vi "MOCKBEAR_Resample.vi"(8 "error in (no error)":errorcluster, 10 "FEA_Model in":refnum<class "FEA_Model.lvclass">, 11 "MOCKBEAR in":refnum<class "MOCKBEAR.lvclass">) -> (0 "error out":errorcluster, 3 "MOCKBEAR out":refnum<class "MOCKBEAR.lvclass">)   [LabVIEW 2021, in "MOCKBEAR.lvclass"]
uses:
  MOCKBEAR.lvclass
  FEA_Model/FEA_Model.lvclass
  MOCKBEAR.lvclass/MOCKBEAR.ctl
panel:
  in  "FFT Window":i32
  in  "New sample rate":dbl
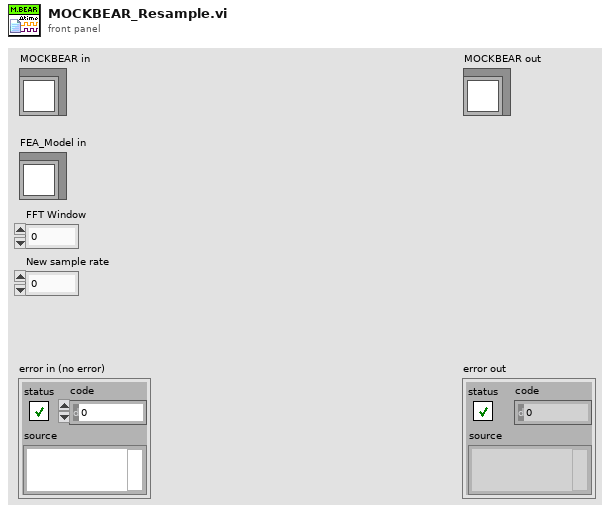
[diagram p1: front panel]
types:
  T1 = enum16{"Recorded", "Auto Resample", "Custom Resample"}
  T2 = cluster{"Modeling Parameters":cluster{"beam_length":dbl, "youngs_modulus":dbl, "torsion_spring":dbl, "beam_height":dbl, "beam_width":dbl, "beam_density":dbl, "number_of_FEA_nodes":i32, "accelerometer_mass":dbl, "M Matrix":dbl[][], "K Matrix":dbl[][], "nodes_of_interest":i32[], "all_nodes":i32[]}, "Simulation Parameters":cluster{"Eigensolver ":enum16{"LabVIEW Cholesky", "LabVIEW General", "LabVIEW Inverse", "LEMP"}, "Pin Estimate":i32, "Frequency Estimate":dbl, "Models Forcasted":i32, "Max frequency":dbl, "Min frequency":dbl, "Frequency delta per node":dbl, "Max frequency delta per second":dbl, "Max Roller Velocity":dbl, "Max Roller Position Percent":dbl, "Min Roller Position Percent":dbl, "Particle Frequencies":dbl[], "Particles":i32[], "Particles Positions":dbl[], "Frequency Target":dbl, "Position estimate":dbl}, "LEMP":cluster{"Eigenvalues":dbl[], "SquareT Eigenvectors":dbl[][], "1/deltaStiff":dbl}}
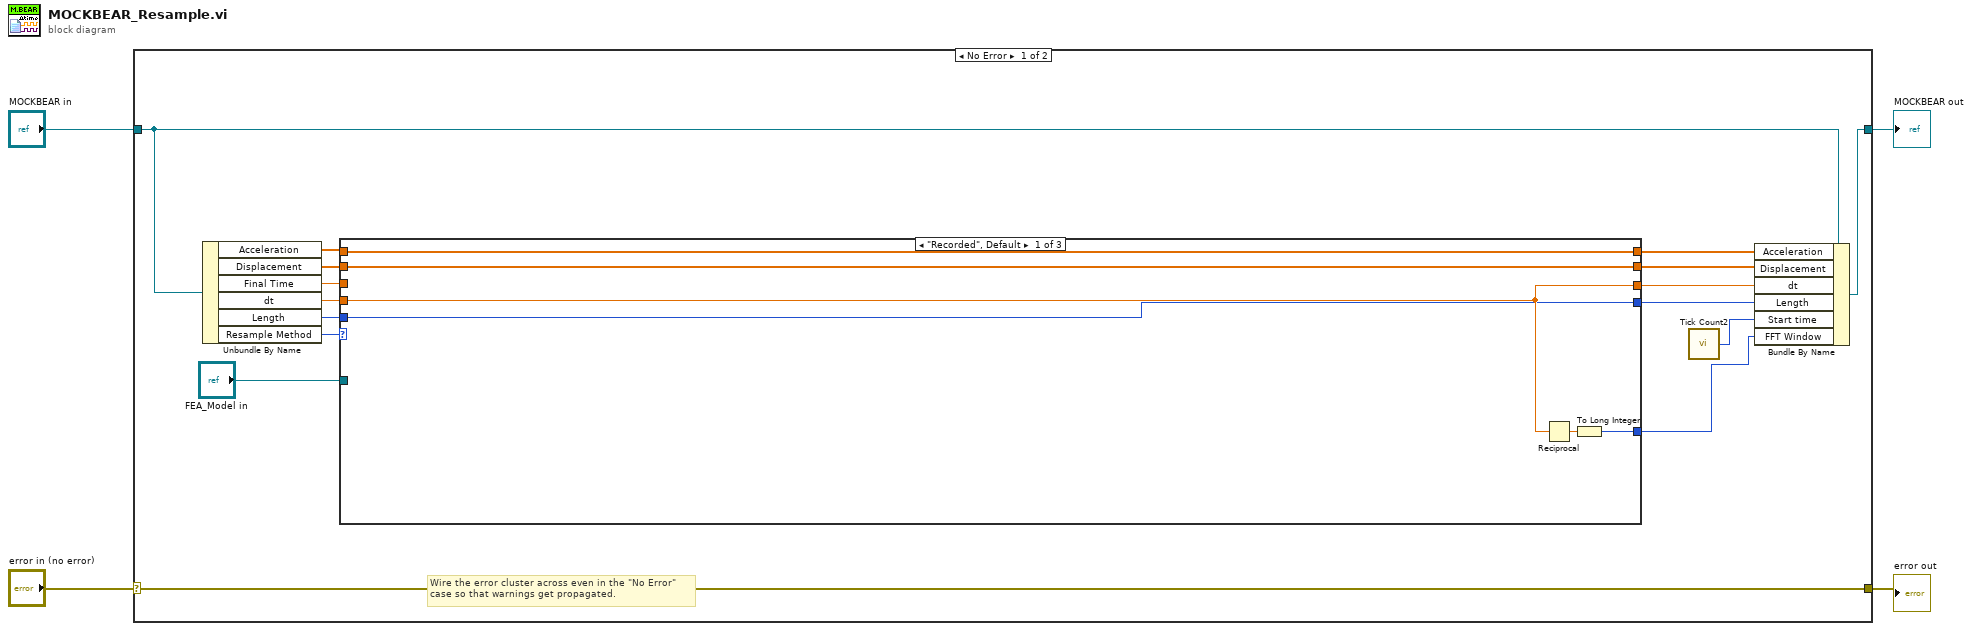
[diagram p0: block diagram]
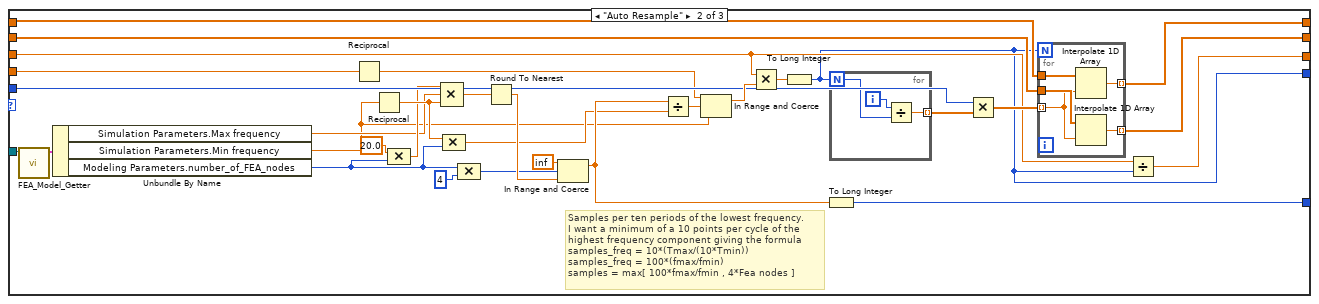
[diagram p2: hidden frame]
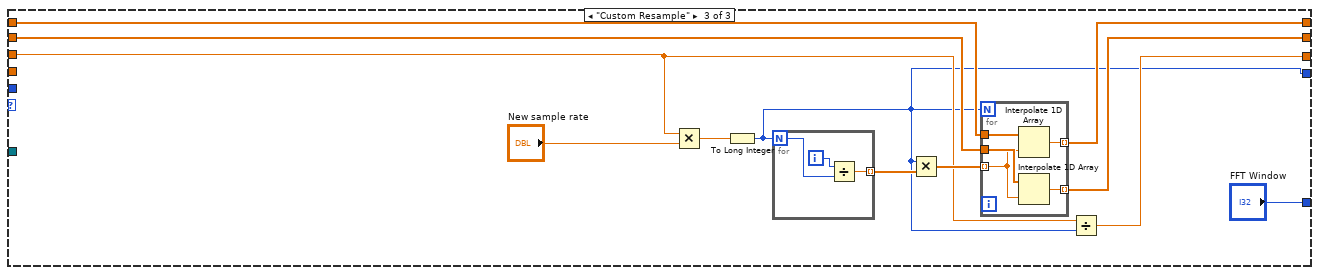
[diagram p3: hidden frame]
diagram:
  n1 = case shown="No Error" "error in (no error)" {
    selector: "error in (no error)" -> [w20 w87]
    tunnel: [w20 w87] -> w3
    tunnel: [w18 w86] -> w1
    tunnel: "MOCKBEAR in" -> [w19 w86]
    frame No Error {
      # "Wire the error cluster across even in the \"No Error\"\ncase so that warnings get propagated."
      n2 = Unbundle By Name(w19) -> ("Acceleration"=w17:dbl[], "Displacement"=w16:dbl[], "Final Time"=w14:dbl, "dt"=w13:dbl, "Length"=w15:i32, "Resample Method"=w12:T1)
      n3 = case shown="\"Recorded\", Default" w12 {
        tunnel: [w24 w54 "FFT Window"] -> w5
        tunnel: [w23 w53 w71] -> w9
        tunnel: [w25 w52 w72] -> w10
        tunnel: [w26 w51 w73] -> w11
        tunnel: w17 -> [w26 w48 w75]
        tunnel: w16 -> [w25 w47 w74]
        tunnel: w15 -> [w22 w46 _]
        tunnel: w14 -> [_ w45 w70]
        tunnel: w13 -> [w23 w44 _]
        tunnel: [w22 w32 w67] -> w7
        tunnel: "FEA_Model in" -> [_ w31 _]
        frame "Recorded", Default {
          n4 = Reciprocal(x=w23) -> (1/x=w21:dbl)
          n5 = To Long Integer(number=w21) -> (32bit integer=w24:i32)
        }
        frame "Auto Resample" {
          # "Samples per ten periods of the lowest frequency. \nI want a minimum of a 10 points per cycle of the \nhighest frequency component giving the formula\nsamples_freq = 10*(Tmax/(10*Tmin)) \nsamples_freq = 100*(fmax/fmin)\nsamples = max[ 100*fmax/fmin , 4*Fea nodes ]"
          n6 = call-dynamic "FEA_Model_Getter.vi"("FEA_Model in"=w31) -> ("FEA Model"=w30:T2)  [unwired: 9 in, 1 out]
          n7 = Unbundle By Name(w30) -> ("Simulation Parameters.Max frequency"=w29:dbl, "Simulation Parameters.Min frequency"=w28:dbl, "Modeling Parameters.number_of_FEA_nodes"=w27:i32)
          n8 = Reciprocal(x=w44) -> (1/x=w33:dbl)
          n9 = Reciprocal(x=w28) -> (1/x=w40:dbl)
          n10 = Compound Arithmetic op=MULTIPLY(20.0 ("value"), w27) -> (w36:dbl)
          n11 = Compound Arithmetic op=MULTIPLY(w36, w29, w40) -> (w43:dbl)
          n12 = Compound Arithmetic op=MULTIPLY(w40, w27) -> (w34:dbl)
          n13 = Compound Arithmetic op=MULTIPLY(w27, 4 ("Modeling Parameters.number_of_FEA_nodes")) -> (w41:i32)
          n14 = Round To Nearest(number=w43) -> (nearest integer value=w42:dbl)
          n15 = In Range and Coerce(upper limit=inf, x=w41, lower limit=w42) -> (coerced(x)=w50:dbl)  [unwired: 1 out]
          n16 = Divide(x=w50, y=w34) -> (x/y=w35:dbl)
          n17 = In Range and Coerce(upper limit=w33, x=w35, lower limit=w28) -> (coerced(x)=w49:dbl)  [unwired: 1 out]
          n18 = Multiply(x=w45, y=w49) -> (x*y=w55:dbl)
          n19 = To Long Integer(number=w55) -> (32bit integer=w32:i32)
          n20 = To Long Integer(number=w50) -> (32bit integer=w54:i32)
          n21 = for {
            N: w32 -> [w59]
            tunnel: [w58] -> w57 mode=indexing
            i -> [w60]
            n22 = Divide(x=w60, y=w59) -> (x/y=w58:dbl)
          }
          n23 = Multiply(x=w46, y=w57) -> (x*y=w56:dbl[])
          n24 = for {
            N: w32 -> [_]
            tunnel: w48 -> [w65]
            tunnel: w47 -> [w64]
            tunnel: w56 -> [w63] mode=indexing
            tunnel: [w62] -> w51 mode=indexing
            tunnel: [w61] -> w52 mode=indexing
            n25 = Interpolate 1D Array(1:w63, 2:w65) -> (0:w62:dbl)
            n26 = Interpolate 1D Array(1:w63, 2:w64) -> (0:w61:dbl)
          }
          n27 = Divide(x=w45, y=w32) -> (x/y=w53:dbl)
        }
        frame "Custom Resample" {
          n28 = Multiply(x=w70, y="New sample rate") -> (x*y=w68:dbl)
          n29 = To Long Integer(number=w68) -> (32bit integer=w67:i32)
          n30 = for {
            N: w67 -> [w79]
            tunnel: [w78] -> w77 mode=indexing
            i -> [w80]
            n31 = Divide(x=w80, y=w79) -> (x/y=w78:dbl)
          }
          n32 = Multiply(x=w67, y=w77) -> (x*y=w76:dbl[])
          n33 = for {
            N: w67 -> [_]
            tunnel: w75 -> [w85]
            tunnel: w74 -> [w84]
            tunnel: w76 -> [w83] mode=indexing
            tunnel: [w82] -> w73 mode=indexing
            tunnel: [w81] -> w72 mode=indexing
            n34 = Interpolate 1D Array(1:w83, 2:w85) -> (0:w82:dbl)
            n35 = Interpolate 1D Array(1:w83, 2:w84) -> (0:w81:dbl)
          }
          n36 = Divide(x=w70, y=w67) -> (x/y=w71:dbl)
        }
      }
      n37 = call "Tick Count2"() -> ("Tick Count(uSec)"=w8:u32)
      n38 = Bundle By Name(cluster=w19, "Acceleration"=w11, "Displacement"=w10, "dt"=w9, "Length"=w7, "Start time"=w8, "FFT Window"=w5) -> (w18:refnum<class "MOCKBEAR.lvclass">)
    }
    frame Error {
    }
  }
  "error out" <- w3
  "MOCKBEAR out" <- w1
